vi "Global_val.vi"() -> ()   [LabVIEW 2018]
panel:
  out "log_Path":path
  in  "move_scale":u16
  in  "Mode":bool
  in  "move_step":dbl=0.03
  in  "start":bool
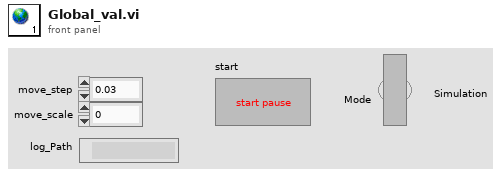
[diagram p1: front panel]
diagram:
